vi "Build Table Definitions.vi"(8 "error in (no error)":errorcluster, 10 "MeasType":T1, 11 "Table Def In":variant) -> (0 "error out":errorcluster, 3 "Table Def Out":variant)   [LabVIEW 2012]
uses:
  Custom Ctrls/ge_MeasType.ctl
  SubVIs Table/Custom Ctls Table/ge_ColDef.ctl
  Controls/HeaderNames.ctl
  SubVIs Table/Custom Ctls Table/ge_HdrInfo.ctl
  SubVIs Table/Custom Ctls Table/ge_GlblCtrls.ctl
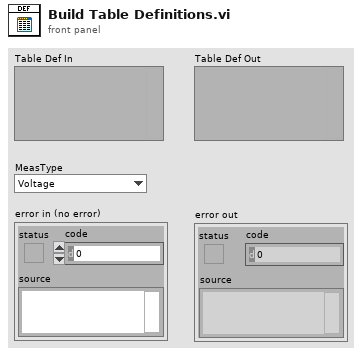
[diagram p1: front panel]
types:
  T1 = typedef "ge_MeasType.ctl" = enum16{"Voltage", "Frequency", "Tachometer", "Dynamic", "Thermocouple", "RTD", "Strain", "Current", "Resistance"}
  T2 = typedef "HeaderNames.ctl" = enum16{"Channel", "Device", "Spacer", "Description", "MB", "Range", "Terminal", "Coupling", "Thresh (V)", "Pulse/Rev", "Slope", "Min EU", "Min RPM", "mV/EU", "Iex", "Temp Units", "Type", "CJC Src", "CJC Val", "Ro", "Wire Cfg", "Strain Mode", "Vex", "Bridge Type", "GF", "Gauge Res", "Poisson", "Lead Res", "Init Strain", "GAF", "Scale", "Offset", "Unit (EU)", "dB?", "dB Ref", "Cal Mag", "Cal Units", "Max Temp", "Min Temp", "Max Strain", "Min Strain"}
  T3 = typedef "ge_GlblCtrls.ctl" = enum16{"Str0", "Bool0", "Bool1", "Int0", "Ring0", "Ring1", "Ring2", "Ring3", "Dbl0", "Dbl1", "Dbl2", "Dbl3", "Cal0", "Cal1", "Cal2", "None"}
  T4 = typedef "ge_ColDef.ctl" = cluster{"ge_HdrNames":T2, "HdrInfo":T5}
  T5 = typedef "ge_HdrInfo.ctl" = cluster{"Hdr Width":i32, "Glbl Ctrl":T3}
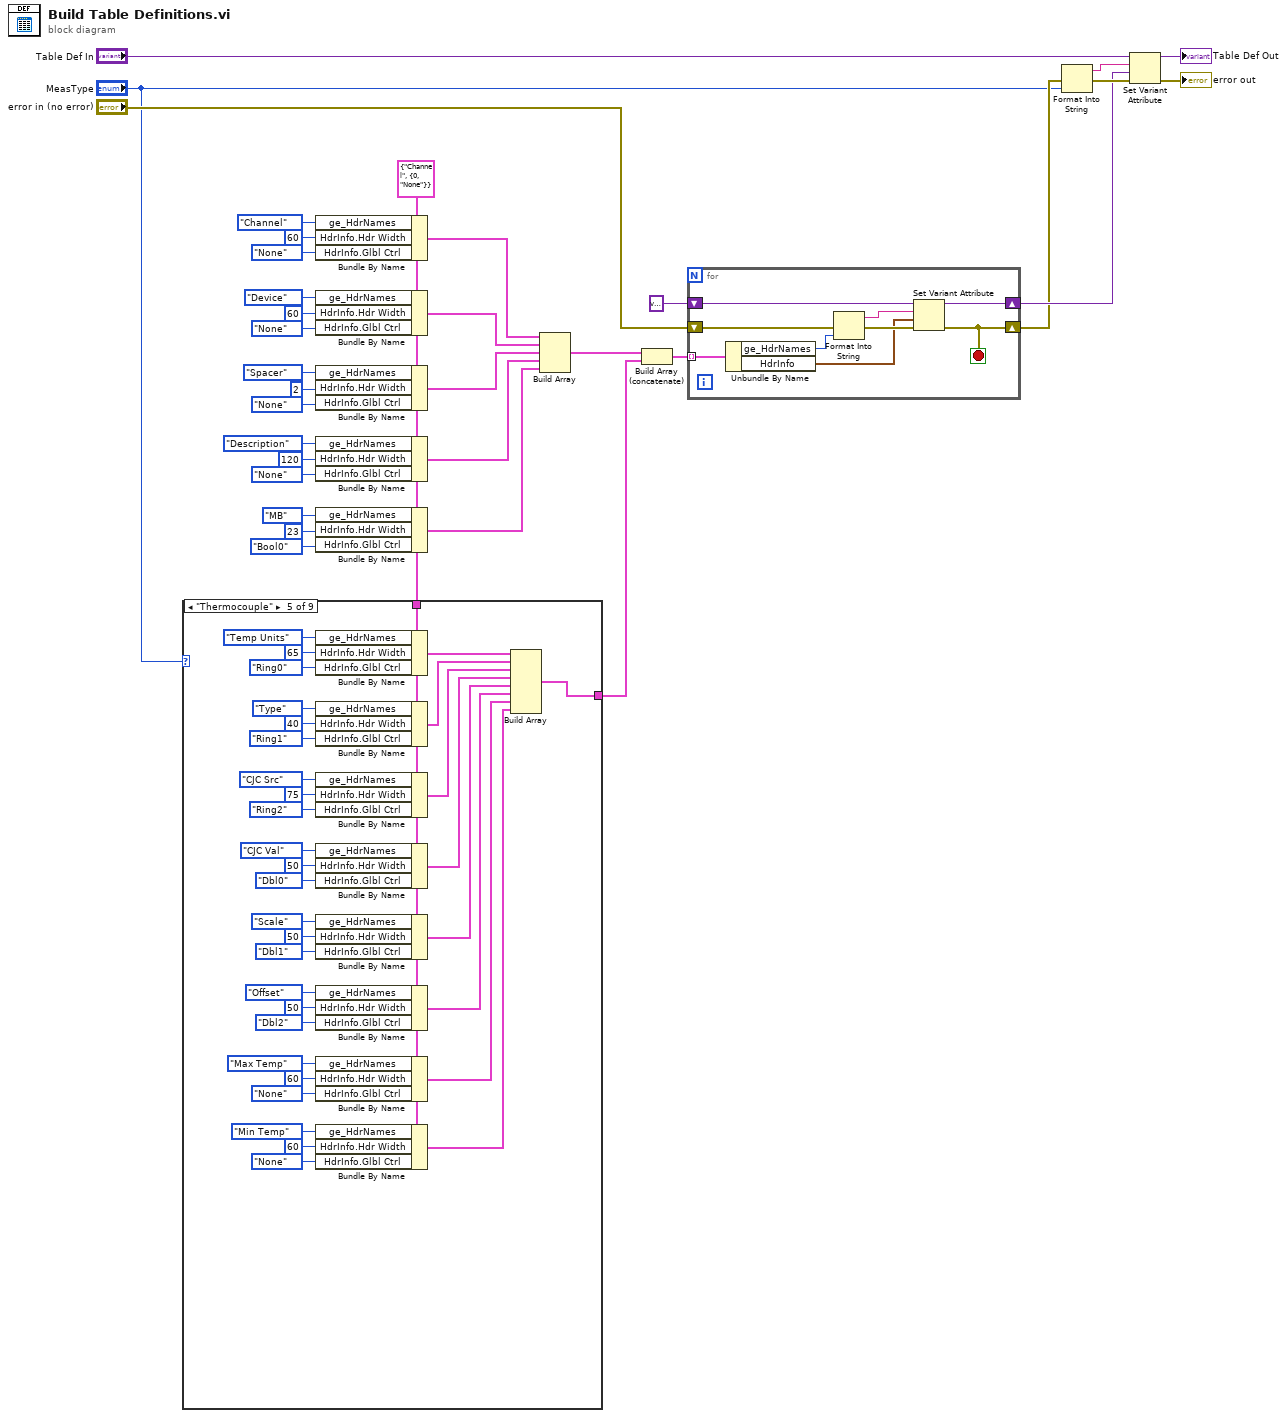
[diagram p0: block diagram]
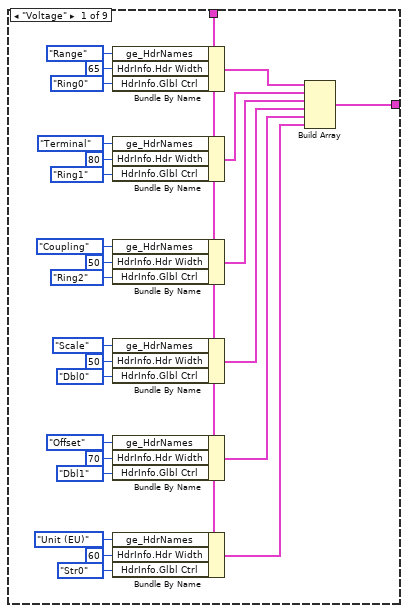
[diagram p2: hidden frame]
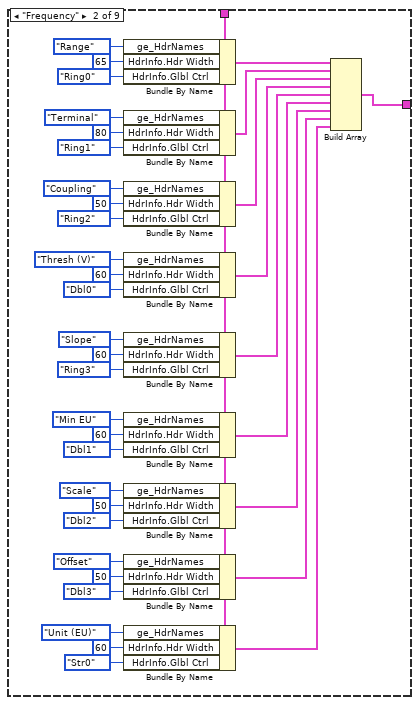
[diagram p3: hidden frame]
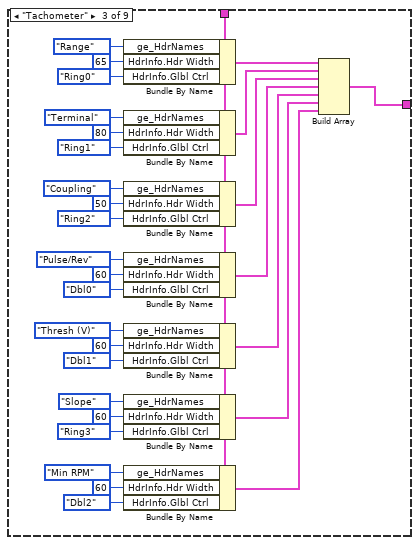
[diagram p4: hidden frame]
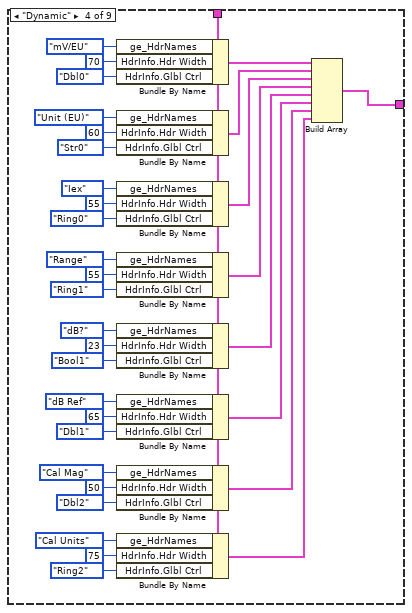
[diagram p5: hidden frame]
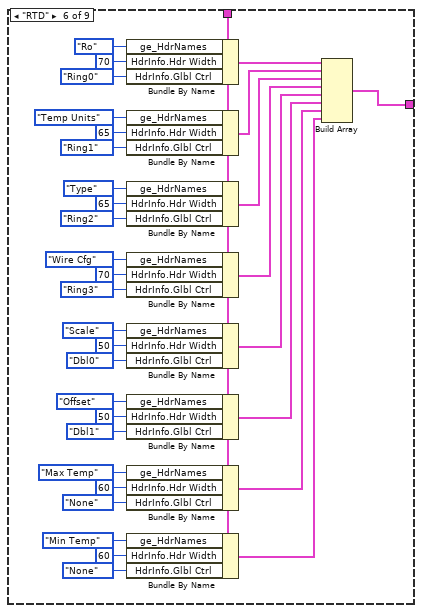
[diagram p6: hidden frame]
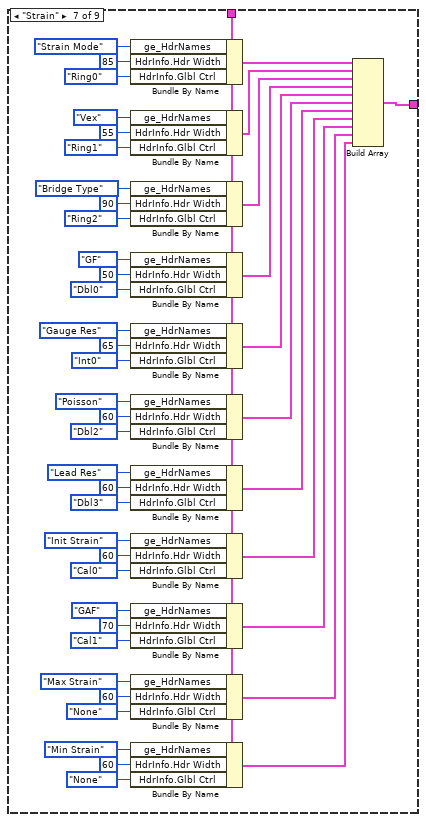
[diagram p7: hidden frame]
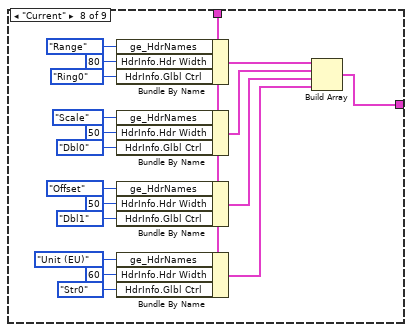
[diagram p8: hidden frame]
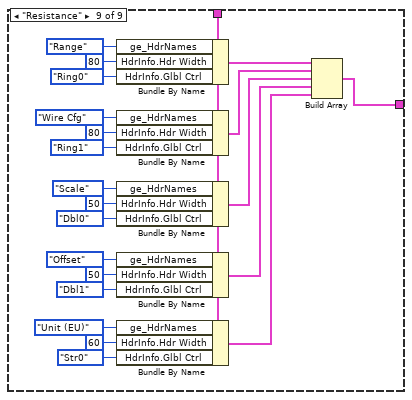
[diagram p9: hidden frame]
diagram:
  w23 = T4 {"ge_HdrNames"=enum."Channel", "HdrInfo"={"Hdr Width"=0, "Glbl Ctrl"=enum."None"}} ("ColDef")
  n1 = case shown="\"Thermocouple\"" "MeasType" {
    tunnel: w23 -> [w58 w63 w100 w130 w164 w198 w232 w277 w296]
    tunnel: [w41 w75 w104 w138 w172 w206 w252 w278 w300] -> w16
    frame "Voltage" {
      n2 = Bundle By Name(cluster=w58, "ge_HdrNames"=HeaderNames."Range", "HdrInfo.Hdr Width"=65, "HdrInfo.Glbl Ctrl"=ge_GlblCtrls."Ring0") -> (w47:T4)
      n3 = Bundle By Name(cluster=w58, "ge_HdrNames"=HeaderNames."Terminal", "HdrInfo.Hdr Width"=80, "HdrInfo.Glbl Ctrl"=ge_GlblCtrls."Ring1") -> (w46:T4)
      n4 = Bundle By Name(cluster=w58, "ge_HdrNames"=HeaderNames."Coupling", "HdrInfo.Hdr Width"=50, "HdrInfo.Glbl Ctrl"=ge_GlblCtrls."Ring2") -> (w45:T4)
      n5 = Bundle By Name(cluster=w58, "ge_HdrNames"=HeaderNames."Scale", "HdrInfo.Hdr Width"=50, "HdrInfo.Glbl Ctrl"=ge_GlblCtrls."Dbl0") -> (w44:T4)
      n6 = Bundle By Name(cluster=w58, "ge_HdrNames"=HeaderNames."Offset", "HdrInfo.Hdr Width"=70, "HdrInfo.Glbl Ctrl"=ge_GlblCtrls."Dbl1") -> (w43:T4)
      n7 = Bundle By Name(cluster=w58, "ge_HdrNames"=HeaderNames."Unit (EU)", "HdrInfo.Hdr Width"=60, "HdrInfo.Glbl Ctrl"=ge_GlblCtrls."Str0") -> (w42:T4)
      n8 = Build Array(w47, w46, w45, w44, w43, w42) -> (w41:T4[])
    }
    frame "Frequency" {
      n9 = Bundle By Name(cluster=w63, "ge_HdrNames"=HeaderNames."Range", "HdrInfo.Hdr Width"=65, "HdrInfo.Glbl Ctrl"=ge_GlblCtrls."Ring0") -> (w80:T4)
      n10 = Bundle By Name(cluster=w63, "ge_HdrNames"=HeaderNames."Terminal", "HdrInfo.Hdr Width"=80, "HdrInfo.Glbl Ctrl"=ge_GlblCtrls."Ring1") -> (w79:T4)
      n11 = Bundle By Name(cluster=w63, "ge_HdrNames"=HeaderNames."Coupling", "HdrInfo.Hdr Width"=50, "HdrInfo.Glbl Ctrl"=ge_GlblCtrls."Ring2") -> (w78:T4)
      n12 = Bundle By Name(cluster=w63, "ge_HdrNames"=HeaderNames."Thresh (V)", "HdrInfo.Hdr Width"=60, "HdrInfo.Glbl Ctrl"=ge_GlblCtrls."Dbl0") -> (w77:T4)
      n13 = Bundle By Name(cluster=w63, "ge_HdrNames"=HeaderNames."Slope", "HdrInfo.Hdr Width"=60, "HdrInfo.Glbl Ctrl"=ge_GlblCtrls."Ring3") -> (w61:T4)
      n14 = Bundle By Name(cluster=w63, "ge_HdrNames"=HeaderNames."Min EU", "HdrInfo.Hdr Width"=60, "HdrInfo.Glbl Ctrl"=ge_GlblCtrls."Dbl1") -> (w62:T4)
      n15 = Bundle By Name(cluster=w63, "ge_HdrNames"=HeaderNames."Scale", "HdrInfo.Hdr Width"=50, "HdrInfo.Glbl Ctrl"=ge_GlblCtrls."Dbl2") -> (w76:T4)
      n16 = Bundle By Name(cluster=w63, "ge_HdrNames"=HeaderNames."Offset", "HdrInfo.Hdr Width"=50, "HdrInfo.Glbl Ctrl"=ge_GlblCtrls."Dbl3") -> (w68:T4)
      n17 = Bundle By Name(cluster=w63, "ge_HdrNames"=HeaderNames."Unit (EU)", "HdrInfo.Hdr Width"=60, "HdrInfo.Glbl Ctrl"=ge_GlblCtrls."Str0") -> (w67:T4)
      n18 = Build Array(w80, w79, w78, w77, w61, w62, w76, w68, w67) -> (w75:T4[])
    }
    frame "Tachometer" {
      n19 = Bundle By Name(cluster=w100, "ge_HdrNames"=HeaderNames."Range", "HdrInfo.Hdr Width"=65, "HdrInfo.Glbl Ctrl"=ge_GlblCtrls."Ring0") -> (w110:T4)
      n20 = Bundle By Name(cluster=w100, "ge_HdrNames"=HeaderNames."Terminal", "HdrInfo.Hdr Width"=80, "HdrInfo.Glbl Ctrl"=ge_GlblCtrls."Ring1") -> (w109:T4)
      n21 = Bundle By Name(cluster=w100, "ge_HdrNames"=HeaderNames."Coupling", "HdrInfo.Hdr Width"=50, "HdrInfo.Glbl Ctrl"=ge_GlblCtrls."Ring2") -> (w108:T4)
      n22 = Bundle By Name(cluster=w100, "ge_HdrNames"=HeaderNames."Pulse/Rev", "HdrInfo.Hdr Width"=60, "HdrInfo.Glbl Ctrl"=ge_GlblCtrls."Dbl0") -> (w107:T4)
      n23 = Bundle By Name(cluster=w100, "ge_HdrNames"=HeaderNames."Thresh (V)", "HdrInfo.Hdr Width"=60, "HdrInfo.Glbl Ctrl"=ge_GlblCtrls."Dbl1") -> (w106:T4)
      n24 = Bundle By Name(cluster=w100, "ge_HdrNames"=HeaderNames."Slope", "HdrInfo.Hdr Width"=60, "HdrInfo.Glbl Ctrl"=ge_GlblCtrls."Ring3") -> (w105:T4)
      n25 = Bundle By Name(cluster=w100, "ge_HdrNames"=HeaderNames."Min RPM", "HdrInfo.Hdr Width"=60, "HdrInfo.Glbl Ctrl"=ge_GlblCtrls."Dbl2") -> (w99:T4)
      n26 = Build Array(w110, w109, w108, w107, w106, w105, w99) -> (w104:T4[])
    }
    frame "Dynamic" {
      n27 = Bundle By Name(cluster=w130, "ge_HdrNames"=HeaderNames."mV/EU", "HdrInfo.Hdr Width"=70, "HdrInfo.Glbl Ctrl"=ge_GlblCtrls."Dbl0") -> (w144:T4)
      n28 = Bundle By Name(cluster=w130, "ge_HdrNames"=HeaderNames."Unit (EU)", "HdrInfo.Hdr Width"=60, "HdrInfo.Glbl Ctrl"=ge_GlblCtrls."Str0") -> (w143:T4)
      n29 = Bundle By Name(cluster=w130, "ge_HdrNames"=HeaderNames."Iex", "HdrInfo.Hdr Width"=55, "HdrInfo.Glbl Ctrl"=ge_GlblCtrls."Ring0") -> (w142:T4)
      n30 = Bundle By Name(cluster=w130, "ge_HdrNames"=HeaderNames."Range", "HdrInfo.Hdr Width"=55, "HdrInfo.Glbl Ctrl"=ge_GlblCtrls."Ring1") -> (w141:T4)
      n31 = Bundle By Name(cluster=w130, "ge_HdrNames"=HeaderNames."dB?", "HdrInfo.Hdr Width"=23, "HdrInfo.Glbl Ctrl"=ge_GlblCtrls."Bool1") -> (w140:T4)
      n32 = Bundle By Name(cluster=w130, "ge_HdrNames"=HeaderNames."dB Ref", "HdrInfo.Hdr Width"=65, "HdrInfo.Glbl Ctrl"=ge_GlblCtrls."Dbl1") -> (w139:T4)
      n33 = Bundle By Name(cluster=w130, "ge_HdrNames"=HeaderNames."Cal Mag", "HdrInfo.Hdr Width"=50, "HdrInfo.Glbl Ctrl"=ge_GlblCtrls."Dbl2") -> (w131:T4)
      n34 = Bundle By Name(cluster=w130, "ge_HdrNames"=HeaderNames."Cal Units", "HdrInfo.Hdr Width"=75, "HdrInfo.Glbl Ctrl"=ge_GlblCtrls."Ring2") -> (w129:T4)
      n35 = Build Array(w144, w143, w142, w141, w140, w139, w131, w129) -> (w138:T4[])
    }
    frame "Thermocouple" {
      n36 = Bundle By Name(cluster=w164, "ge_HdrNames"=HeaderNames."Temp Units", "HdrInfo.Hdr Width"=65, "HdrInfo.Glbl Ctrl"=ge_GlblCtrls."Ring0") -> (w178:T4)
      n37 = Bundle By Name(cluster=w164, "ge_HdrNames"=HeaderNames."Type", "HdrInfo.Hdr Width"=40, "HdrInfo.Glbl Ctrl"=ge_GlblCtrls."Ring1") -> (w177:T4)
      n38 = Bundle By Name(cluster=w164, "ge_HdrNames"=HeaderNames."CJC Src", "HdrInfo.Hdr Width"=75, "HdrInfo.Glbl Ctrl"=ge_GlblCtrls."Ring2") -> (w176:T4)
      n39 = Bundle By Name(cluster=w164, "ge_HdrNames"=HeaderNames."CJC Val", "HdrInfo.Hdr Width"=50, "HdrInfo.Glbl Ctrl"=ge_GlblCtrls."Dbl0") -> (w175:T4)
      n40 = Bundle By Name(cluster=w164, "ge_HdrNames"=HeaderNames."Scale", "HdrInfo.Hdr Width"=50, "HdrInfo.Glbl Ctrl"=ge_GlblCtrls."Dbl1") -> (w174:T4)
      n41 = Bundle By Name(cluster=w164, "ge_HdrNames"=HeaderNames."Offset", "HdrInfo.Hdr Width"=50, "HdrInfo.Glbl Ctrl"=ge_GlblCtrls."Dbl2") -> (w173:T4)
      n42 = Bundle By Name(cluster=w164, "ge_HdrNames"=HeaderNames."Max Temp", "HdrInfo.Hdr Width"=60, "HdrInfo.Glbl Ctrl"=ge_GlblCtrls."None") -> (w165:T4)
      n43 = Bundle By Name(cluster=w164, "ge_HdrNames"=HeaderNames."Min Temp", "HdrInfo.Hdr Width"=60, "HdrInfo.Glbl Ctrl"=ge_GlblCtrls."None") -> (w163:T4)
      n44 = Build Array(w178, w177, w176, w175, w174, w173, w165, w163) -> (w172:T4[])
    }
    frame "RTD" {
      n45 = Bundle By Name(cluster=w198, "ge_HdrNames"=HeaderNames."Ro", "HdrInfo.Hdr Width"=70, "HdrInfo.Glbl Ctrl"=ge_GlblCtrls."Ring0") -> (w212:T4)
      n46 = Bundle By Name(cluster=w198, "ge_HdrNames"=HeaderNames."Temp Units", "HdrInfo.Hdr Width"=65, "HdrInfo.Glbl Ctrl"=ge_GlblCtrls."Ring1") -> (w211:T4)
      n47 = Bundle By Name(cluster=w198, "ge_HdrNames"=HeaderNames."Type", "HdrInfo.Hdr Width"=65, "HdrInfo.Glbl Ctrl"=ge_GlblCtrls."Ring2") -> (w210:T4)
      n48 = Bundle By Name(cluster=w198, "ge_HdrNames"=HeaderNames."Wire Cfg", "HdrInfo.Hdr Width"=70, "HdrInfo.Glbl Ctrl"=ge_GlblCtrls."Ring3") -> (w209:T4)
      n49 = Bundle By Name(cluster=w198, "ge_HdrNames"=HeaderNames."Scale", "HdrInfo.Hdr Width"=50, "HdrInfo.Glbl Ctrl"=ge_GlblCtrls."Dbl0") -> (w208:T4)
      n50 = Bundle By Name(cluster=w198, "ge_HdrNames"=HeaderNames."Offset", "HdrInfo.Hdr Width"=50, "HdrInfo.Glbl Ctrl"=ge_GlblCtrls."Dbl1") -> (w207:T4)
      n51 = Bundle By Name(cluster=w198, "ge_HdrNames"=HeaderNames."Max Temp", "HdrInfo.Hdr Width"=60, "HdrInfo.Glbl Ctrl"=ge_GlblCtrls."None") -> (w199:T4)
      n52 = Bundle By Name(cluster=w198, "ge_HdrNames"=HeaderNames."Min Temp", "HdrInfo.Hdr Width"=60, "HdrInfo.Glbl Ctrl"=ge_GlblCtrls."None") -> (w197:T4)
      n53 = Build Array(w212, w211, w210, w209, w208, w207, w199, w197) -> (w206:T4[])
    }
    frame "Strain" {
      n54 = Bundle By Name(cluster=w232, "ge_HdrNames"=HeaderNames."Strain Mode", "HdrInfo.Hdr Width"=85, "HdrInfo.Glbl Ctrl"=ge_GlblCtrls."Ring0") -> (w258:T4)
      n55 = Bundle By Name(cluster=w232, "ge_HdrNames"=HeaderNames."Vex", "HdrInfo.Hdr Width"=55, "HdrInfo.Glbl Ctrl"=ge_GlblCtrls."Ring1") -> (w257:T4)
      n56 = Bundle By Name(cluster=w232, "ge_HdrNames"=HeaderNames."Bridge Type", "HdrInfo.Hdr Width"=90, "HdrInfo.Glbl Ctrl"=ge_GlblCtrls."Ring2") -> (w256:T4)
      n57 = Bundle By Name(cluster=w232, "ge_HdrNames"=HeaderNames."GF", "HdrInfo.Hdr Width"=50, "HdrInfo.Glbl Ctrl"=ge_GlblCtrls."Dbl0") -> (w255:T4)
      n58 = Bundle By Name(cluster=w232, "ge_HdrNames"=HeaderNames."Gauge Res", "HdrInfo.Hdr Width"=65, "HdrInfo.Glbl Ctrl"=ge_GlblCtrls."Int0") -> (w254:T4)
      n59 = Bundle By Name(cluster=w232, "ge_HdrNames"=HeaderNames."Poisson", "HdrInfo.Hdr Width"=60, "HdrInfo.Glbl Ctrl"=ge_GlblCtrls."Dbl2") -> (w253:T4)
      n60 = Bundle By Name(cluster=w232, "ge_HdrNames"=HeaderNames."Lead Res", "HdrInfo.Hdr Width"=60, "HdrInfo.Glbl Ctrl"=ge_GlblCtrls."Dbl3") -> (w245:T4)
      n61 = Bundle By Name(cluster=w232, "ge_HdrNames"=HeaderNames."Init Strain", "HdrInfo.Hdr Width"=60, "HdrInfo.Glbl Ctrl"=ge_GlblCtrls."Cal0") -> (w244:T4)
      n62 = Bundle By Name(cluster=w232, "ge_HdrNames"=HeaderNames."GAF", "HdrInfo.Hdr Width"=70, "HdrInfo.Glbl Ctrl"=ge_GlblCtrls."Cal1") -> (w234:T4)
      n63 = Bundle By Name(cluster=w232, "ge_HdrNames"=HeaderNames."Max Strain", "HdrInfo.Hdr Width"=60, "HdrInfo.Glbl Ctrl"=ge_GlblCtrls."None") -> (w233:T4)
      n64 = Bundle By Name(cluster=w232, "ge_HdrNames"=HeaderNames."Min Strain", "HdrInfo.Hdr Width"=60, "HdrInfo.Glbl Ctrl"=ge_GlblCtrls."None") -> (w231:T4)
      n65 = Build Array(w258, w257, w256, w255, w254, w253, w245, w244, w234, w233, w231) -> (w252:T4[])
    }
    frame "Current" {
      n66 = Bundle By Name(cluster=w277, "ge_HdrNames"=HeaderNames."Range", "HdrInfo.Hdr Width"=80, "HdrInfo.Glbl Ctrl"=ge_GlblCtrls."Ring0") -> (w282:T4)
      n67 = Bundle By Name(cluster=w277, "ge_HdrNames"=HeaderNames."Scale", "HdrInfo.Hdr Width"=50, "HdrInfo.Glbl Ctrl"=ge_GlblCtrls."Dbl0") -> (w281:T4)
      n68 = Bundle By Name(cluster=w277, "ge_HdrNames"=HeaderNames."Offset", "HdrInfo.Hdr Width"=50, "HdrInfo.Glbl Ctrl"=ge_GlblCtrls."Dbl1") -> (w280:T4)
      n69 = Bundle By Name(cluster=w277, "ge_HdrNames"=HeaderNames."Unit (EU)", "HdrInfo.Hdr Width"=60, "HdrInfo.Glbl Ctrl"=ge_GlblCtrls."Str0") -> (w279:T4)
      n70 = Build Array(w282, w281, w280, w279) -> (w278:T4[])
    }
    frame "Resistance" {
      n71 = Bundle By Name(cluster=w296, "ge_HdrNames"=HeaderNames."Range", "HdrInfo.Hdr Width"=80, "HdrInfo.Glbl Ctrl"=ge_GlblCtrls."Ring0") -> (w304:T4)
      n72 = Bundle By Name(cluster=w296, "ge_HdrNames"=HeaderNames."Wire Cfg", "HdrInfo.Hdr Width"=80, "HdrInfo.Glbl Ctrl"=ge_GlblCtrls."Ring1") -> (w303:T4)
      n73 = Bundle By Name(cluster=w296, "ge_HdrNames"=HeaderNames."Scale", "HdrInfo.Hdr Width"=50, "HdrInfo.Glbl Ctrl"=ge_GlblCtrls."Dbl0") -> (w302:T4)
      n74 = Bundle By Name(cluster=w296, "ge_HdrNames"=HeaderNames."Offset", "HdrInfo.Hdr Width"=50, "HdrInfo.Glbl Ctrl"=ge_GlblCtrls."Dbl1") -> (w301:T4)
      n75 = Bundle By Name(cluster=w296, "ge_HdrNames"=HeaderNames."Unit (EU)", "HdrInfo.Hdr Width"=60, "HdrInfo.Glbl Ctrl"=ge_GlblCtrls."Str0") -> (w295:T4)
      n76 = Build Array(w304, w303, w302, w301, w295) -> (w300:T4[])
    }
  }
  n77 = Bundle By Name(cluster=w23, "ge_HdrNames"=HeaderNames."Channel", "HdrInfo.Hdr Width"=60, "HdrInfo.Glbl Ctrl"=ge_GlblCtrls."None") -> (w22:T4)
  n78 = Bundle By Name(cluster=w23, "ge_HdrNames"=HeaderNames."Device", "HdrInfo.Hdr Width"=60, "HdrInfo.Glbl Ctrl"=ge_GlblCtrls."None") -> (w21:T4)
  n79 = Bundle By Name(cluster=w23, "ge_HdrNames"=HeaderNames."Spacer", "HdrInfo.Hdr Width"=2, "HdrInfo.Glbl Ctrl"=ge_GlblCtrls."None") -> (w20:T4)
  n80 = Bundle By Name(cluster=w23, "ge_HdrNames"=HeaderNames."Description", "HdrInfo.Hdr Width"=120, "HdrInfo.Glbl Ctrl"=ge_GlblCtrls."None") -> (w19:T4)
  n81 = Bundle By Name(cluster=w23, "ge_HdrNames"=HeaderNames."MB", "HdrInfo.Hdr Width"=23, "HdrInfo.Glbl Ctrl"=ge_GlblCtrls."Bool0") -> (w18:T4)
  n82 = Build Array(w22, w21, w20, w19, w18) -> (w17:T4[])
  n83 = Build Array (concatenate)(w17, w16) -> (w15:T4[])
  n84 = for {
    tunnel: w15 -> [w325] mode=indexing
    shift-right: [w319] -> w11
    shift-left: variant ("variant") -> [w320]
    shift-right: [w317] -> w10
    shift-left: "error in (no error)" -> [w318]
    stop <- w317 stop-if-true
    n85 = Unbundle By Name(w325) -> ("ge_HdrNames"=w322:T2, "HdrInfo"=w321:T5)
    n86 = Format Into String(error in=w318, w322) -> (resulting string=w324:string, error out=w323:errorcluster)  [unwired: 2 in]
    n87 = Set Variant Attribute(Variant=w320, name=w324, value=w321, error in=w323) -> (Variant out=w319:variant, error out=w317:errorcluster)  [unwired: 1 out]
  }
  n88 = Format Into String(error in=w10, "MeasType") -> (resulting string=w12:string, error out=w13:errorcluster)  [unwired: 2 in]
  n89 = Set Variant Attribute(Variant="Table Def In", name=w12, value=w11, error in=w13) -> (Variant out=→"Table Def Out":variant, error out=→"error out":errorcluster)  [unwired: 1 out]
